vi "rechst weiter.vi"(8 "error in (no error)":errorcluster caption="Fehler (Eingang, kein Fehler)", 11 "Device ID":T1(ring)) -> (0 "error out":errorcluster caption="Fehler (Ausgang)", 2 "geradeaus?":bool, 3 "Device ID Out":T1(ring))   [LabVIEW 2010]
uses:
  globale Variable 1.vi
panel:
  out "Aktuelle Position":i32
  in  "pneumatik?":bool
  in  "ende?":bool
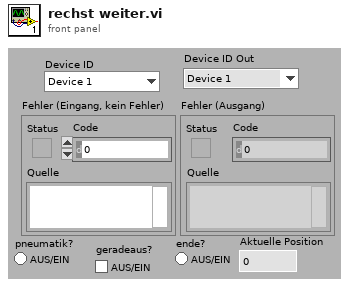
[diagram p1: front panel]
types:
  T1 = enum16{"Device 1", "Device 2", "Device 3", "Device 4", "Device 5", "Device 6", "Device 7", "Device 8"}
  T2 = enum8{"Output 1 (O1)", "Output 2 (O2)", "Output 3 (O3)", "Output 4 (O4)", "Output 5 (O5)", "Output 6 (O6)", "Output 7 (O7)", "Output 8 (O8)"}
  T3 = enum8{"Robo Interface", "Extension 1", "Extension 2", "Extension 3"}
  T4 = enum8{"Power 1", "Power 2", "Power 3", "Power 4", "Power 5", "Power 6", "Power 7", "Power 8"}
  T5 = enum8{"Input 1 (I1)", "Input 2 (I2)", "Input 3 (I3)", "Input 4 (I4)", "Input 5 (I5)", "Input 6 (I6)", "Input 7 (I7)", "Input 8 (I8)"}
  T6 = enum8{"Goes High", "Goes Low", "Goes High or Low"}
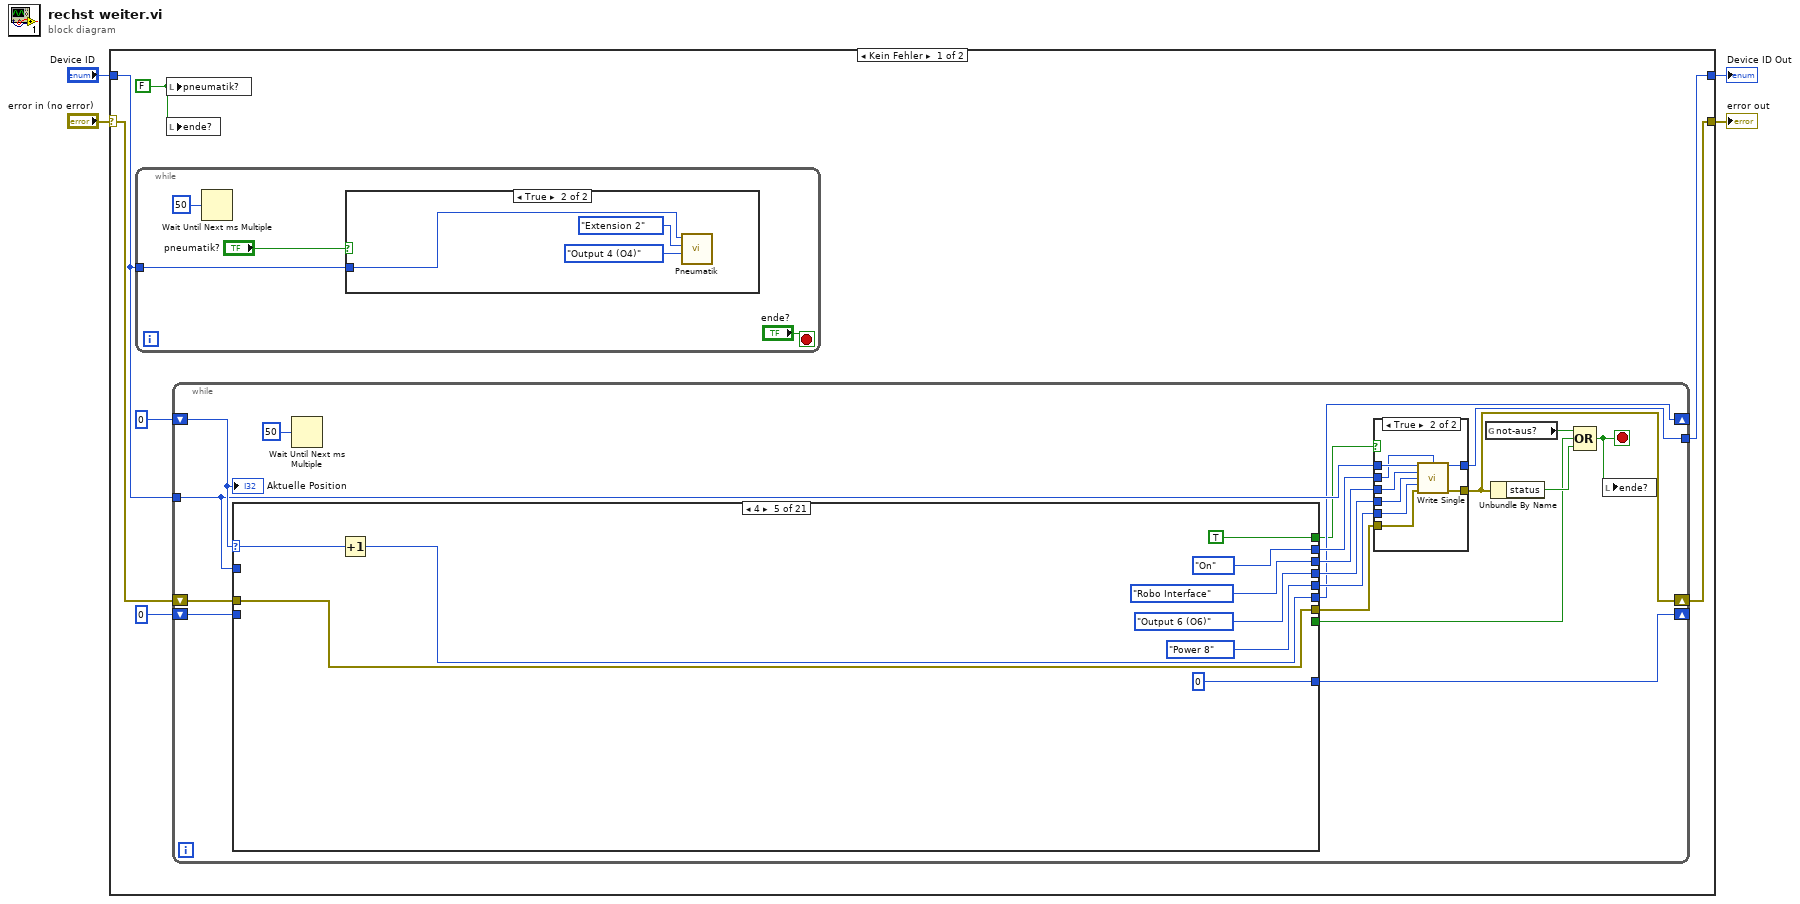
[diagram p0: block diagram]
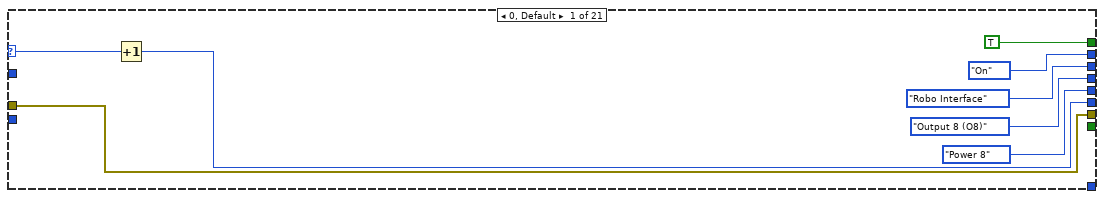
[diagram p3: hidden frame]
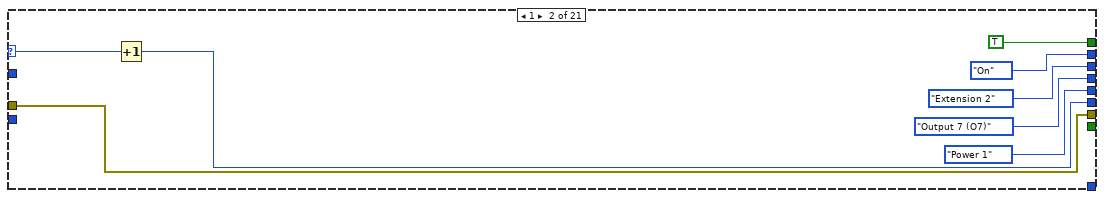
[diagram p4: hidden frame]
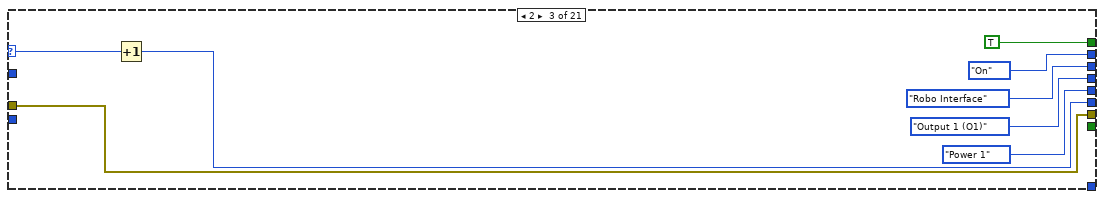
[diagram p5: hidden frame]
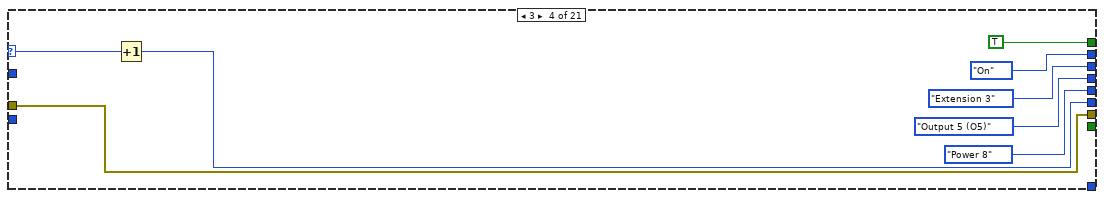
[diagram p6: hidden frame]
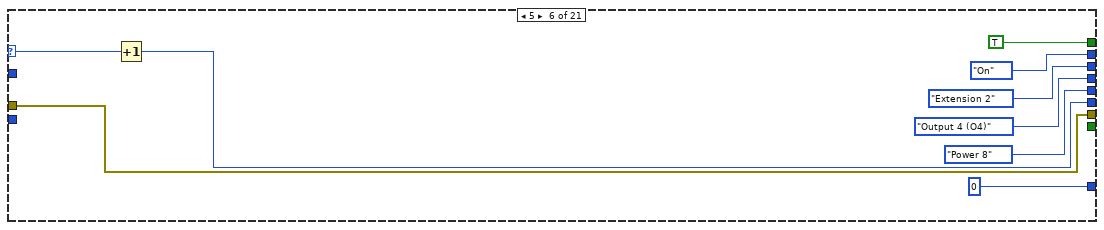
[diagram p7: hidden frame]
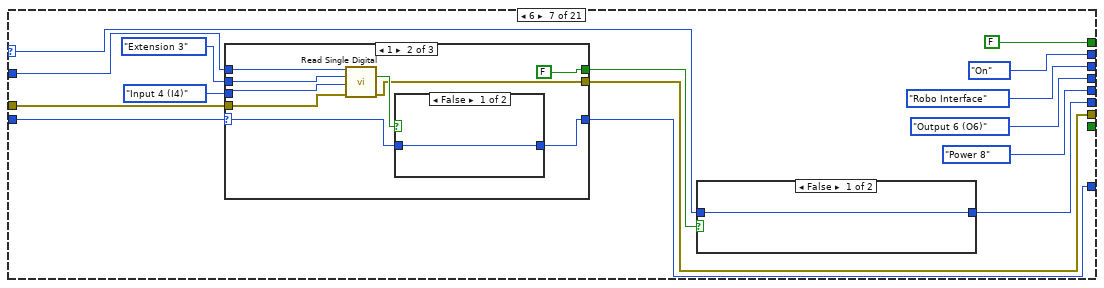
[diagram p8: hidden frame]
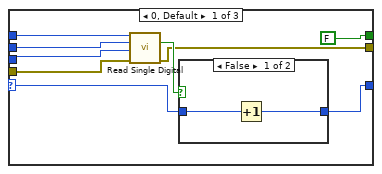
[diagram p9: hidden frame]
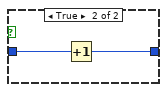
[diagram p11: hidden frame]
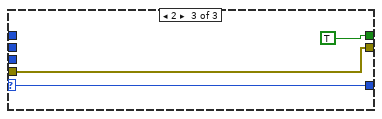
[diagram p12: hidden frame]
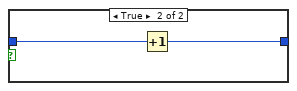
[diagram p13: hidden frame]
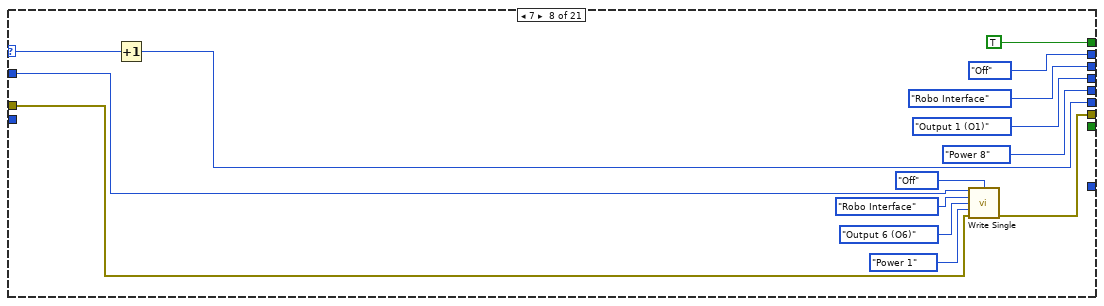
[diagram p14: hidden frame]
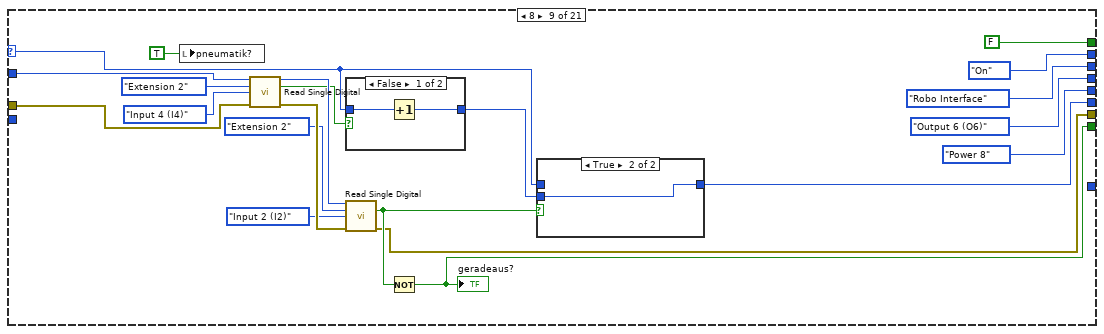
[diagram p15: hidden frame]
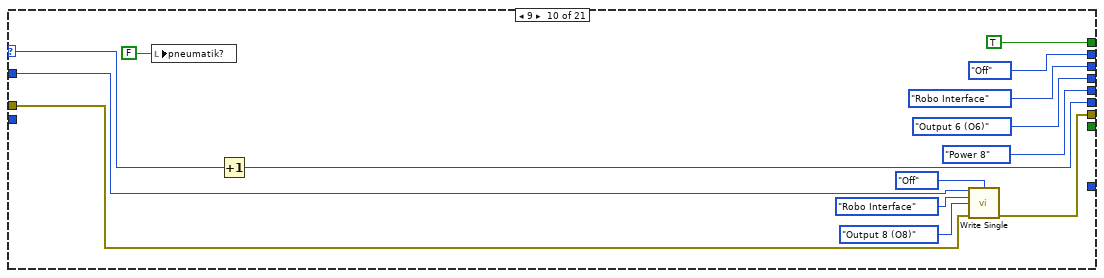
[diagram p18: hidden frame]
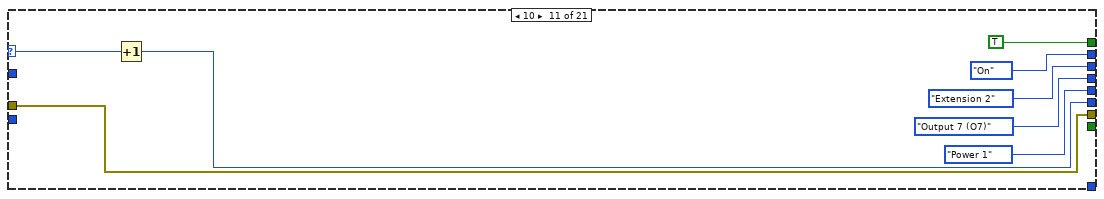
[diagram p19: hidden frame]
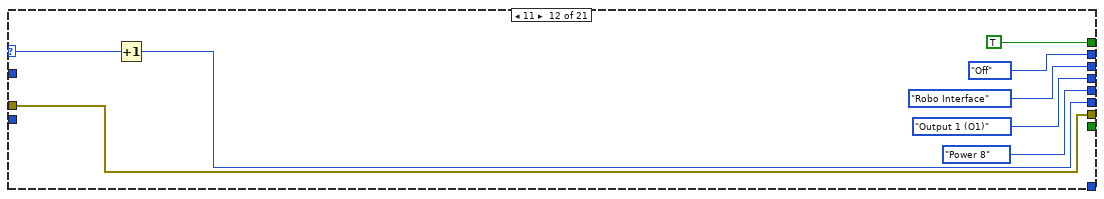
[diagram p20: hidden frame]
diagram:
  n1 = case shown="Kein Fehler" "error in (no error)" {
    selector: "error in (no error)" -> [w10 w304]
    tunnel: [w9 w304] -> w3
    tunnel: [w8 w303] -> w2
    tunnel: "Device ID" -> [w6 w303]
    frame No Error {
      w5 = FALSE ("pneumatik?")
      n2 = while {
        tunnel: w6 -> [w12]
        stop <- "ende?" stop-if-true
        n3 = Wait Until Next ms Multiple(millisecond multiple=50) -> ()  [unwired: 1 out]
        n4 = case shown="TRUE" "pneumatik?" {
          tunnel: w12 -> [_ w16]
          frame False {
          }
          frame True {
            n5 = call "Pneumatik.vi"("Single_Output"=T2."Output 4 (O4)", "Module"=T3."Extension 2", "Device ID"=w16) -> ()  [unwired: 1 in, 8 out]
          }
        }
      }
      n6 = local write "pneumatik?"(w5) -> ()
      n7 = local write "ende?"(w5) -> ()
      n8 = while {
        shift-right: [w21] -> _
        shift-left: 0 -> [w31]
        shift-right: [w35] -> w9
        shift-left: w10 -> [w28]
        tunnel: [w36] -> w8
        tunnel: w6 -> [w30]
        shift-right: [w20] -> _
        shift-left: 0 -> [w29]
        stop <- w32 stop-if-true
        n9 = case shown="4" w31 {
          selector: w31 -> [w39 w47 w55 w63 w73 w82 w97 w140 w152 w180 w188 w196 w204 w212 w233 w240 w253 w261 w270 w279 w287]
          tunnel: [TRUE ("AN/Aus") TRUE ("AN/Aus") TRUE ("AN/Aus") TRUE ("AN/Aus") TRUE ("AN/Aus") TRUE ("AN/Aus") FALSE ("AN/Aus") TRUE ("AN/Aus") FALSE ("AN/Aus") TRUE ("AN/Aus") TRUE ("AN/Aus") TRUE ("AN/Aus") TRUE ("AN/Aus") TRUE ("AN/Aus") FALSE ("AN/Aus") TRUE ("AN/Aus") FALSE ("AN/Aus") TRUE ("AN/Aus") FALSE ("AN/Aus") TRUE ("AN/Aus") FALSE ("AN/Aus")] -> w19
          tunnel: [enum8{"Off", "On"}."On" ("Output_Action") enum8{"Off", "On"}."On" ("Output_Action") enum8{"Off", "On"}."On" ("Output_Action") enum8{"Off", "On"}."On" ("Output_Action") enum8{"Off", "On"}."On" ("Output_Action") enum8{"Off", "On"}."On" ("Output_Action") enum8{"Off", "On"}."On" ("Output_Action") enum8{"Off", "On"}."Off" ("Output_Action") enum8{"Off", "On"}."On" ("Output_Action") enum8{"Off", "On"}."Off" ("Output_Action") enum8{"Off", "On"}."On" ("Output_Action") enum8{"Off", "On"}."Off" ("Output_Action") enum8{"Off", "On"}."On" ("Output_Action") enum8{"Off", "On"}."Off" ("Output_Action") enum8{"Off", "On"}."Off" ("Output_Action") enum8{"Off", "On"}."Off" ("Output_Action") enum8{"Off", "On"}."Off" ("Output_Action") enum8{"Off", "On"}."Off" ("Output_Action") enum8{"Off", "On"}."Off" ("Output_Action") enum8{"Off", "On"}."Off" ("Output_Action") enum8{"Off", "On"}."Off" ("Output_Action")] -> w27
          tunnel: [T2."Output 8 (O8)" ("Single_Output") T2."Output 7 (O7)" ("Single_Output") T2."Output 1 (O1)" ("Single_Output") T2."Output 5 (O5)" ("Single_Output") T2."Output 6 (O6)" ("Single_Output") T2."Output 4 (O4)" ("Single_Output") T2."Output 6 (O6)" ("Single_Output") T2."Output 1 (O1)" ("Single_Output") T2."Output 6 (O6)" ("Single_Output") T2."Output 6 (O6)" ("Single_Output") T2."Output 7 (O7)" ("Single_Output") T2."Output 1 (O1)" ("Single_Output") T2."Output 8 (O8)" ("Single_Output") T2."Output 5 (O5)" ("Single_Output") T2."Output 1 (O1)" ("Single_Output") T2."Output 7 (O7)" ("Single_Output") T2."Output 6 (O6)" ("Single_Output") T2."Output 8 (O8)" ("Single_Output") T2."Output 7 (O7)" ("Single_Output") T2."Output 8 (O8)" ("Single_Output") T2."Output 6 (O6)" ("Single_Output")] -> w25
          tunnel: [T4."Power 8" ("Output_PWM") T4."Power 1" ("Output_PWM") T4."Power 1" ("Output_PWM") T4."Power 8" ("Output_PWM") T4."Power 8" ("Output_PWM") T4."Power 8" ("Output_PWM") T4."Power 8" ("Output_PWM") T4."Power 8" ("Output_PWM") T4."Power 8" ("Output_PWM") T4."Power 8" ("Output_PWM") T4."Power 1" ("Output_PWM") T4."Power 8" ("Output_PWM") T4."Power 8" ("Output_PWM") T4."Power 8" ("Output_PWM") T4."Power 8" ("Output_PWM") T4."Power 8" ("Output_PWM") T4."Power 8" ("Output_PWM") T4."Power 8" ("Output_PWM") T4."Power 8" ("Output_PWM") T4."Power 8" ("Output_PWM") T4."Power 8" ("Output_PWM")] -> w24
          tunnel: [T3."Robo Interface" ("Module") T3."Extension 2" ("Module") T3."Robo Interface" ("Module") T3."Extension 3" ("Module") T3."Robo Interface" ("Module") T3."Extension 2" ("Module") T3."Robo Interface" ("Module") T3."Robo Interface" ("Module") T3."Robo Interface" ("Module") T3."Robo Interface" ("Module") T3."Extension 2" ("Module") T3."Robo Interface" ("Module") T3."Extension 2" ("Module") T3."Extension 3" ("Module") T3."Robo Interface" ("Module") T3."Extension 2" ("Module") T3."Extension 2" ("Module") T3."Robo Interface" ("Module") T3."Extension 2" ("Module") T3."Extension 2" ("Module") T3."Extension 2" ("Module")] -> w26
          tunnel: w30 -> [_ _ _ _ _ _ w95 w139 w154 w175 _ _ _ _ w232 _ w252 _ _ _ _]
          tunnel: w28 -> [w40 w48 w56 w64 w70 w79 w88 w138 w153 w174 w187 w195 w203 w211 w229 w241 w251 w260 w269 w278 w286]
          tunnel: [w40 w48 w56 w64 w70 w79 w94 w133 w149 w173 w187 w195 w203 w211 w226 w241 w250 w260 w269 w278 w286] -> w23
          tunnel: [w38 w46 w54 w62 w72 w81 w96 w141 w156 w181 w189 w197 w205 w213 w234 w242 w254 w262 w268 w276 w287] -> w21
          tunnel: w29 -> [_ _ _ _ _ _ w92 _ _ _ _ _ _ _ _ _ _ _ _ _ _]
          tunnel: [_ _ _ _ 0 0 w89 _ _ _ _ _ _ _ _ _ _ _ _ _ _] -> w20
          tunnel: [_ _ _ _ _ _ _ _ w147 _ _ _ _ _ _ _ _ _ _ FALSE TRUE] -> w22
          frame 0, Default {
            n10 = Increment(x=w39) -> (x+1=w38:i32)
          }
          frame 1 {
            n11 = Increment(x=w47) -> (x+1=w46:i32)
          }
          frame 2 {
            n12 = Increment(x=w55) -> (x+1=w54:i32)
          }
          frame 3 {
            n13 = Increment(x=w63) -> (x+1=w62:i32)
          }
          frame 4 {
            n14 = Increment(x=w73) -> (x+1=w72:i32)
          }
          frame 5 {
            n15 = Increment(x=w82) -> (x+1=w81:i32)
          }
          frame 6 {
            n16 = case shown="1" w92 {
              selector: w92 -> [w110 w122 w128]
              tunnel: w95 -> [w106 w117 _]
              tunnel: w88 -> [w105 w118 w127]
              tunnel: [w103 w115 w127] -> w94
              tunnel: [FALSE ("Value") FALSE ("Value") TRUE ("Value")] -> w93
              tunnel: T3."Extension 3" ("Module") -> [w107 w120 _]
              tunnel: T5."Input 4 (I4)" ("Digital_Input") -> [w108 w119 _]
              tunnel: [w109 w121 w128] -> w89
              frame 0, Default {
                n17 = call "Read Single Digital.vi"("Device ID"=w106, "Module"=w107, "Digital_Input"=w108, "error in"=w105) -> ("Value"=w104:bool, "error out"=w103:errorcluster)  [unwired: 10 out]
                n18 = case shown="FALSE" w104 {
                  tunnel: w110 -> [w113 w114]
                  tunnel: [w112 w114] -> w109
                  frame False {
                    n19 = Increment(x=w113) -> (x+1=w112:i32)
                  }
                  frame True {
                  }
                }
              }
              frame 1 {
                n20 = call "Read Single Digital.vi"("Device ID"=w117, "Module"=w120, "Digital_Input"=w119, "error in"=w118) -> ("Value"=w116:bool, "error out"=w115:errorcluster)  [unwired: 10 out]
                n21 = case shown="FALSE" w116 {
                  tunnel: w122 -> [w124 w126]
                  tunnel: [w124 w125] -> w121
                  frame False {
                  }
                  frame True {
                    n22 = Increment(x=w126) -> (x+1=w125:i32)
                  }
                }
              }
              frame 2 {
              }
            }
            n23 = case shown="FALSE" w93 {
              tunnel: w97 -> [w130 w132]
              tunnel: [w130 w131] -> w96
              frame False {
              }
              frame True {
                n24 = Increment(x=w132) -> (x+1=w131:i32)
              }
            }
          }
          frame 7 {
            n25 = Increment(x=w140) -> (x+1=w141:i32)
            n26 = call "Write Single.vi"("Device ID"=w139, "Output_Action"=enum8{"Off", "On"}."Off", "Module"=T3."Robo Interface", "Single_Output"=T2."Output 6 (O6)", "Output_PWM"=T4."Power 1", "error in"=w138) -> ("error out"=w133:errorcluster)  [unwired: 9 out]
          }
          frame 8 {
            n27 = local write "pneumatik?"(TRUE ("pneumatik?")) -> ()
            n28 = call "Read Single Digital.vi"("Device ID"=w154, "Module"=T3."Extension 2", "Digital_Input"=T5."Input 4 (I4)", "error in"=w153) -> ("Device ID Out"=w161:T1, "Value"=w155:bool, "error out"=w160:errorcluster)  [unwired: 9 out]
            n29 = case shown="FALSE" w155 {
              tunnel: w152 -> [w169 w170]
              tunnel: [w168 w170] -> w157
              frame False {
                n30 = Increment(x=w169) -> (x+1=w168:i32)
              }
              frame True {
              }
            }
            n31 = call "Read Single Digital.vi"("Device ID"=w161, "Module"=T3."Extension 2", "Digital_Input"=T5."Input 2 (I2)", "error in"=w160) -> ("Value"=w151:bool, "error out"=w149:errorcluster)  [unwired: 10 out]
            n32 = Not(x=w151) -> (.not. x?=w147:bool)
            "geradeaus?" <- w147
            n33 = case shown="TRUE" w151 {
              tunnel: w157 -> [_ w172]
              tunnel: [w171 w172] -> w156
              tunnel: w152 -> [w171 _]
              frame False {
              }
              frame True {
              }
            }
          }
          frame 9 {
            n34 = local write "pneumatik?"(FALSE ("pneumatik?")) -> ()
            n35 = Increment(x=w180) -> (x+1=w181:i32)
            n36 = call "Write Single.vi"("Device ID"=w175, "Output_Action"=enum8{"Off", "On"}."Off", "Module"=T3."Robo Interface", "Single_Output"=T2."Output 8 (O8)", "error in"=w174) -> ("error out"=w173:errorcluster)  [unwired: 1 in, 9 out]
          }
          frame 10 {
            n37 = Increment(x=w188) -> (x+1=w189:i32)
          }
          frame 11 {
            n38 = Increment(x=w196) -> (x+1=w197:i32)
          }
          frame 12 {
            n39 = Increment(x=w204) -> (x+1=w205:i32)
          }
          frame 13 {
            n40 = Increment(x=w212) -> (x+1=w213:i32)
          }
          frame 14 {
            n41 = Increment(x=w233) -> (x+1=w234:i32)
            n42 = call "Wait Until Digital Edge.vi"("Device ID"=w232, "Wait Until"=T6."Goes High", "Module"=T3."Extension 2", "Digital_Input"=T5."Input 3 (I3)", "error in"=w229, "Time Out (10)"=inf) -> ("Device ID Out"=w225:T1, "error out"=w220:errorcluster)  [unwired: 8 out]
            n43 = call "Write Single.vi"("Device ID"=w225, "Output_Action"=enum8{"Off", "On"}."On", "Module"=T3."Robo Interface", "Single_Output"=T2."Output 8 (O8)", "Output_PWM"=T4."Power 8", "error in"=w220) -> ("error out"=w219:errorcluster)  [unwired: 9 out]
            n44 = call "Verzögerung"("error in (no error)"=w219) -> ("error out"=w226:errorcluster)  [unwired: 1 in, 9 out]
          }
          frame 15 {
            n45 = Increment(x=w240) -> (x+1=w242:i32)
          }
          frame 16 {
            n46 = Increment(x=w253) -> (x+1=w254:i32)
            n47 = call "Pneumatik.vi"("error in (no error)"=w251, "Single_Output"=T2."Output 3 (O3)", "Module"=T3."Extension 2", "Device ID"=w252) -> ("error out"=w250:errorcluster)  [unwired: 7 out]
          }
          frame 17 {
            n48 = Increment(x=w261) -> (x+1=w262:i32)
          }
          frame 18 {
            n49 = Increment(x=w270) -> (x+1=w268:i32)
          }
          frame 19 {
            n50 = Increment(x=w279) -> (x+1=w276:i32)
          }
          frame 20 {
          }
        }
        n51 = Wait Until Next ms Multiple(millisecond multiple=50) -> ()  [unwired: 1 out]
        n52 = case shown="TRUE" w19 {
          tunnel: w30 -> [w294 w302]
          tunnel: [w293 w301] -> w35
          tunnel: [w294 w300] -> w36
          tunnel: w27 -> [_ w299]
          tunnel: w26 -> [_ w298]
          tunnel: w25 -> [_ w297]
          tunnel: w24 -> [_ w296]
          tunnel: w23 -> [w293 w295]
          frame False {
          }
          frame True {
            n53 = call "Write Single.vi"("Device ID"=w302, "Output_Action"=w299, "Module"=w298, "Single_Output"=w297, "Output_PWM"=w296, "error in"=w295) -> ("Device ID Out"=w300:T1, "error out"=w301:errorcluster)  [unwired: 8 out]
          }
        }
        n54 = global read "globale Variable 1.vi" "not-aus?"() -> (w33:bool)
        n55 = Unbundle By Name(w35) -> ("status"=w34:bool)
        n56 = Compound Arithmetic op=OR(w33, w22, w34) -> (w32:bool)
        n57 = local write "ende?"(w32) -> ()
        "Aktuelle Position" <- w31
      }
    }
    frame Error {
    }
  }
  "error out" <- w3
  "Device ID Out" <- w2
